vi "User_log_read_write.vi"(8 "error in":errorcluster, 10 "Action":string="Begin", 11 "User":string="Joe") -> (0 "error out":errorcluster)   [LabVIEW 2016]
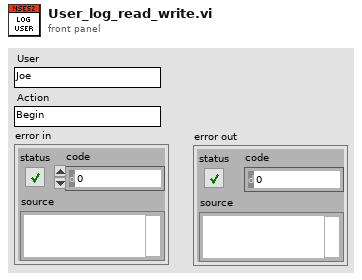
[diagram p1: front panel]
types:
  T1 = enum16{"open", "replace", "create", "open or create", "replace or create", "replace or create with confirmation"}
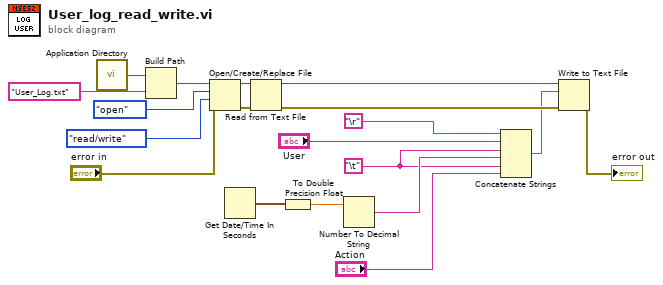
[diagram p0: block diagram]
diagram:
  w6 = "\t"
  n1 = call <vilib>:"Application Directory.vi"() -> ("Application Directory"=w19:path)
  n2 = Build Path(base path=w19, name or relative path="User_Log.txt") -> (appended path=w13:path)
  n3 = Open/Create/Replace File(file path (use dialog)=w13, error in="error in", operation (0:open)=T1."open", access (0:read/write)=enum16{"read/write", "read-only", "write-only"}."read/write") -> (refnum out=w12:refnum<file>, error out=w3:errorcluster)  [unwired: 2 in, 1 out]
  n4 = Get Date/Time In Seconds() -> (seconds since 1Jan1904=w9:timestamp)
  n5 = Read from Text File(file (use dialog)=w12, error in=w3) -> (refnum out=w17:refnum<file>, error out=w16:errorcluster)  [unwired: 2 in, 2 out]
  n6 = To Double Precision Float(number=w9) -> (double precision float=w8:dbl)
  n7 = Number To Decimal String(number=w8) -> (decimal integer string=w7:string)  [unwired: 1 in]
  n8 = Concatenate Strings("\r", "User", w6, w7, w6, "Action") -> (w15:string)
  n9 = Write to Text File(file (use dialog)=w17, text=w15, error in=w16) -> (error out=→"error out":errorcluster)  [unwired: 1 in, 2 out]
